vi "Wrap.vi"(7 "Actor in":refnum<class "Actor.lvclass">, 8 "Error in":errorcluster, 10 "Msg DVR in":refnum<data-value>, 11 "Msg in":refnum<class "Msg.lvclass">) -> (0 "Error out":errorcluster, 2 "Msg DVR out":refnum<data-value>, 5 "Actor out":refnum<class "Actor.lvclass">)   [LabVIEW 2020, in "jettl.lvlib" / "Msg.lvclass"]
uses:
  Msg.lvclass
  Actor/Actor.lvclass
  Msg Contents/Msg Contents.lvclass
  Unified Actor Relation.ctl
  jettl.lvlib
  Teller.ctl
  Msg.ctl
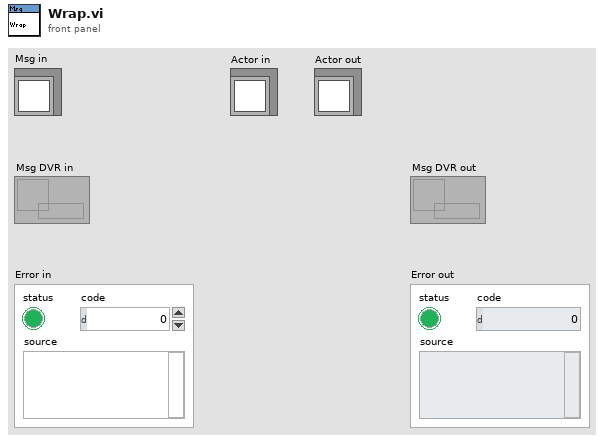
[diagram p1: front panel]
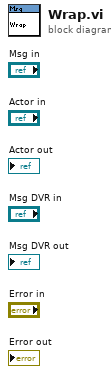
[diagram p0: block diagram]
diagram:
